vi "GenBlackKeyDataArray.vi"(5 "BlackKeySize":cluster{"Width":i32, "Hieght":i32}={"Width"=10, "Hieght"=97}, 8 "error in (no error)":errorcluster) -> (0 "error out":errorcluster, 2 "BlackKeyData array":u32[][](array[numeric]))   [LabVIEW 2015]
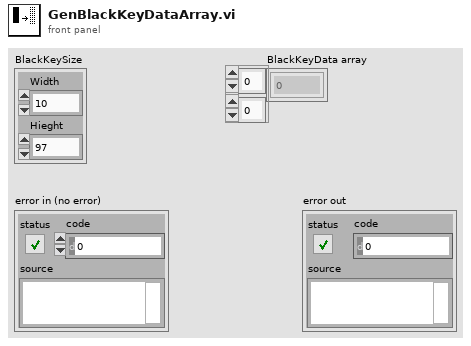
[diagram p1: front panel]
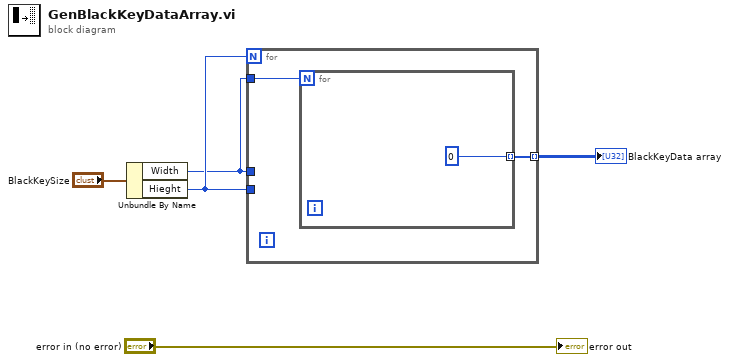
[diagram p0: block diagram]
diagram:
  n1 = Unbundle By Name("BlackKeySize") -> ("Width"=w4:i32, "Hieght"=w5:i32)
  n2 = for {
    N: w5 -> [_]
    tunnel: w4 -> [_]
    tunnel: w5 -> [_]
    tunnel: [w7] -> w2 mode=indexing
    tunnel: w4 -> [w6]
    n3 = for {
      N: w6 -> [_]
      tunnel: [u32 0] -> w7 mode=indexing
    }
  }
  "BlackKeyData array" <- w2
  "error out" <- "error in (no error)"
